vi "zero_Padder.vi"(10 "facteur de résolution fréquentielle":i32, 11 "Graphe en entrée":waveform(dbl) caption="Graphe") -> (3 "Graphe en sortie":waveform(dbl) caption="Graphe")   [LabVIEW 2024]
uses:
  <vilib>/Waveform/WDTOps.llb/WDT Number of Waveform Samples DBL.vi
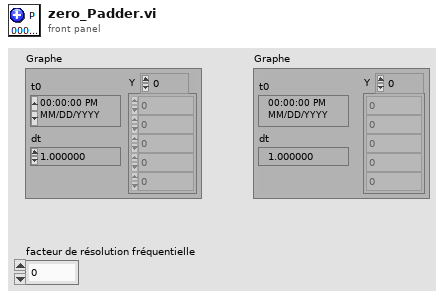
[diagram p1: front panel]
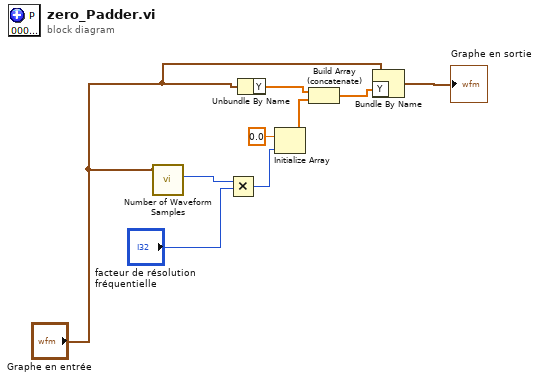
[diagram p0: block diagram]
diagram:
  n1 = call-poly <vilib>:"Number of Waveform Samples.vi"("waveform in"="Graphe en entrée") -> ("number of samples"=w7:i32)  [unwired: 8 in, 2 out]
  n2 = Multiply(x=w7, y="facteur de résolution fréquentielle") -> (x*y=w8:i32)
  n3 = Unbundle By Name("Graphe en entrée") -> ("Y"=w1:dbl[])
  n4 = Initialize Array(0.0 ("élément"), w8) -> (w3:dbl[])
  n5 = Build Array (concatenate)(w1, w3) -> (w4:dbl[])
  n6 = Bundle By Name(cluster="Graphe en entrée", "Y"=w4) -> (→"Graphe en sortie":waveform(dbl))
